vi "Main.vi"(8 "error in (no error)":errorcluster, 11 "StageSPIMBase in":refnum<class "StageSPIM.lvclass">) -> (0 "error out":errorcluster, 3 "component":refnum<class "StageSPIM.lvclass">)   [LabVIEW 2012, in "StageSPIM.lvclass"]
doc: "Main VI of the component."
uses:
  StageSPIM.lvclass
  <vilib>/Distrio/Murmex/Murmex/command_enum.ctl
  StageSPIM.lvclass/StageSPIM.ctl
  <vilib>/Distrio/Murmex/InitialiseMessage/InitialiseMessage.lvclass
  <vilib>/Distrio/Murmex/TerminateMessage/TerminateMessage.lvclass
  <vilib>/Distrio/Murmex/Murmex/update_cluster.ctl
  <vilib>/Distrio/Murmex/GenericMessage/GenericMessage.lvclass
  <vilib>/Distrio/Murmex/StopMessage/StopMessage.lvclass
  <vilib>/Distrio/Murmex/ConfigureMessage/ConfigureMessage.lvclass
  Global terminating.vi
  <vilib>/Distrio/Murmex/Murmex/Set configure at initialise.vi
  <vilib>/Distrio/Murmex/Murmex/Set log reference.vi
  <vilib>/Distrio/Murmex/Murmex/Set VI reference.vi
  <vilib>/Distrio/Murmex/Murmex/Get ID.vi
  <vilib>/Distrio/Murmex/Murmex/Set write log to disk.vi
  <vilib>/Distrio/Murmex/Murmex/Murmex.lvclass
  <vilib>/Distrio/Murmex/Message/Message.lvclass
panel:
  in  "Log position?":bool
  in  "button::stop":bool
  in  "button::configure":bool
  in  "button::quit":bool
  in  "Tab Control":enum32{"Main", "Debug"}(tab)
  in  "forwardFocus":bool
  in  "backFocus":bool
  in  "stepFocus":dbl[unit]
  out "currentFocus":dbl[unit]
  in  "speedFocus":dbl[unit]
  in  "targetFocus":dbl[unit]
  in  "forwardY":bool
  in  "backY":bool
  in  "stepY":dbl[unit]
  in  "forwardZ":bool
  in  "backZ":bool
  in  "stepZ":dbl[unit]
  in  "forwardX":bool
  in  "backX":bool
  in  "stepX":dbl[unit]
  in  "forwardA":bool
  in  "backA":bool
  in  "stepA":dbl[unit]
  out "currentA":dbl[unit]
  out "currentX":dbl[unit]
  out "currentY":dbl[unit]
  out "currentZ":dbl[unit]
  in  "speedZ":dbl[unit]
  in  "speedY":dbl[unit]
  in  "speedX":dbl[unit]
  in  "speedA":dbl[unit]
  in  "targetA":dbl[unit]
  in  "targetX":dbl[unit]
  in  "targetY":dbl[unit]
  in  "targetZ":dbl[unit]
  in  "button::send":bool
  out "log":string
  in  "command":T1
  in  "Generic command":string
  in  "ID":string="stage"
  out "terminate?":bool=TRUE
  # "Current\nposition"
  # "Target\nposition"
  # "Steps"
  # "Speed"
  # "A"
  # "X"
  # "Y"
  # "Z"
  # "Focus"
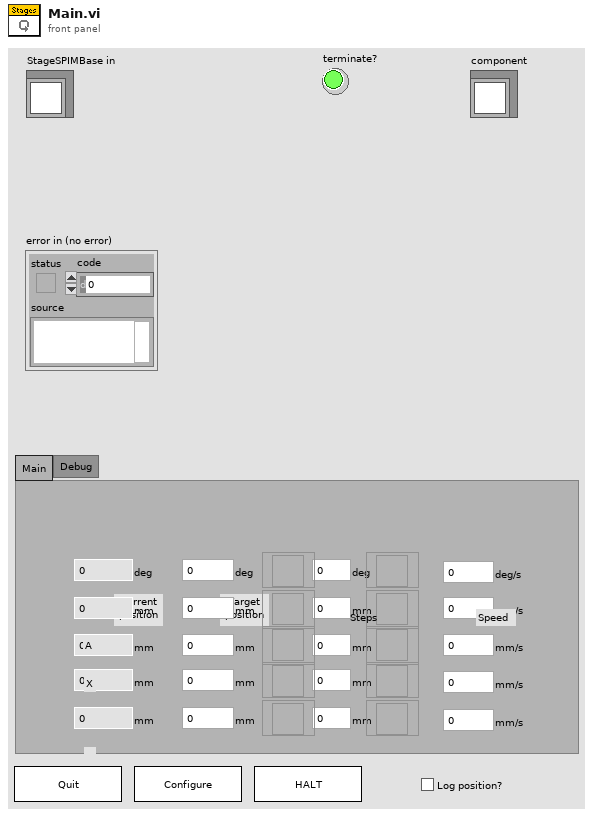
[diagram p1: front panel]
types:
  T1 = typedef "Murmex.lvlib/Murmex.lvclass/command_enum.ctl" = enum16{"null", "initialise", "reset", "terminate", "acknowledge", "update", "inspect", "inform", "proceed", "start", "stop", "fetch", "configure", "generic"}
  T2 = enum8{"Enabled", "Disabled", "Disabled and Grayed Out"}
  T3 = typedef "Murmex.lvlib/Murmex.lvclass/update_cluster.ctl" = cluster{"target ID":string, "key chains":string[], "values":variant[]}
  T4 = typedef "Murmex.lvlib/Murmex.lvclass/Event type enumerations.ctl" = enum16{"before", "after"}
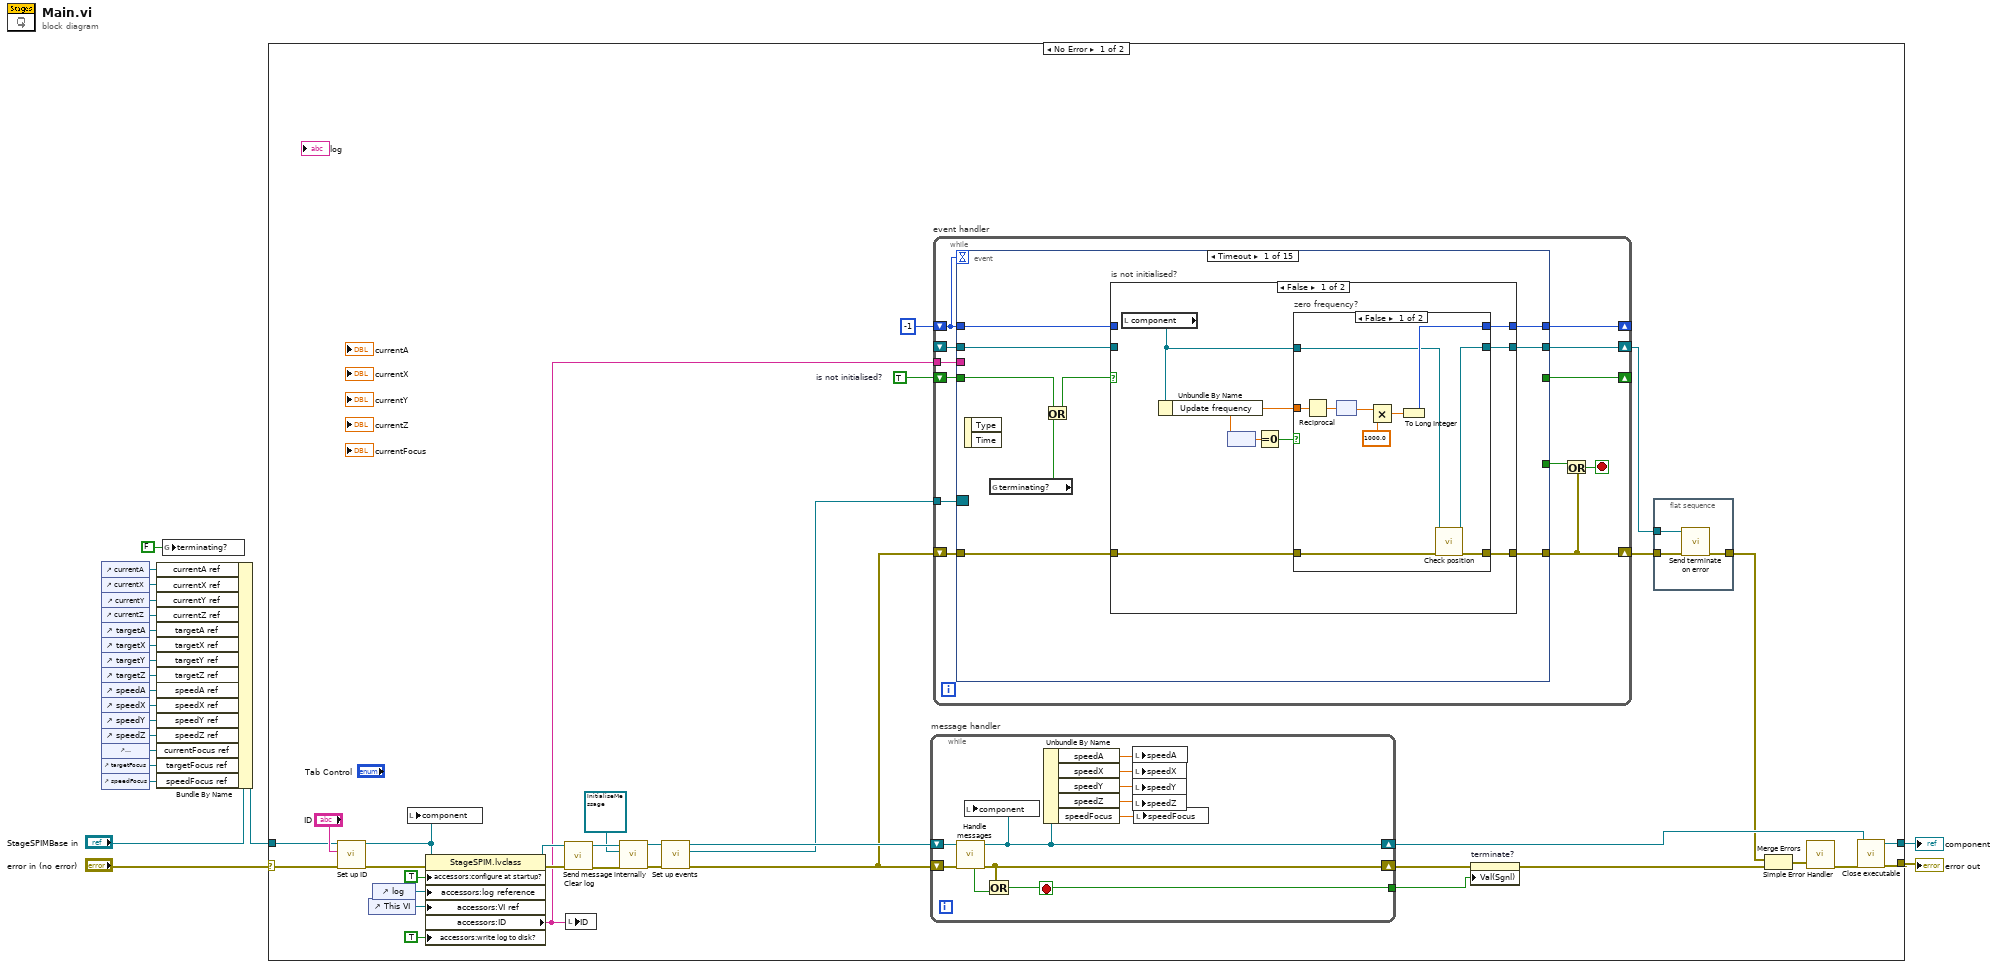
[diagram p0: block diagram]
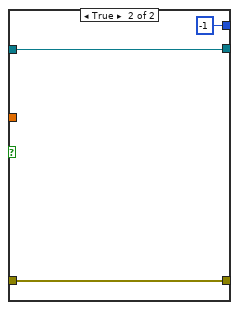
[diagram p2: hidden frame]
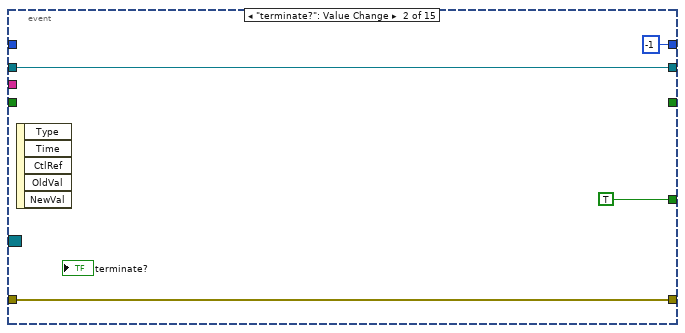
[diagram p4: hidden frame]
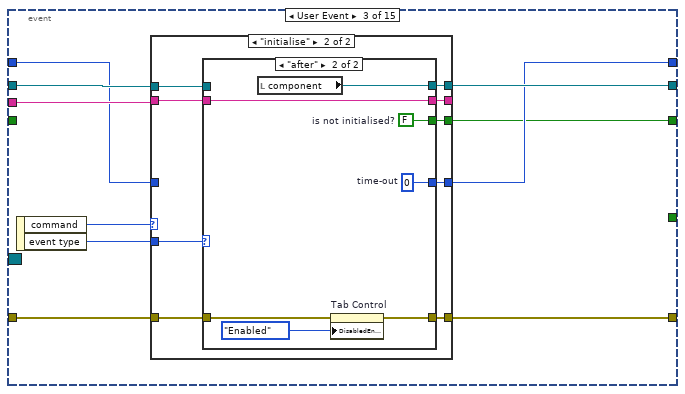
[diagram p5: hidden frame]
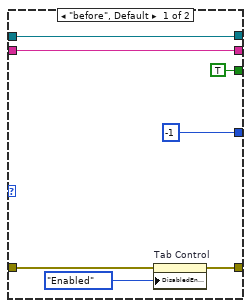
[diagram p7: hidden frame]
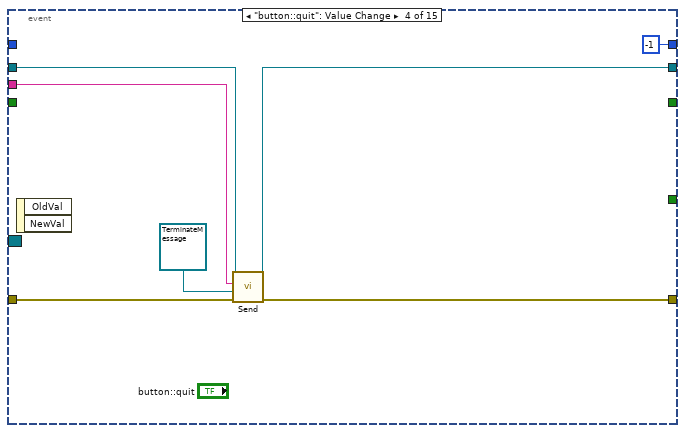
[diagram p8: hidden frame]
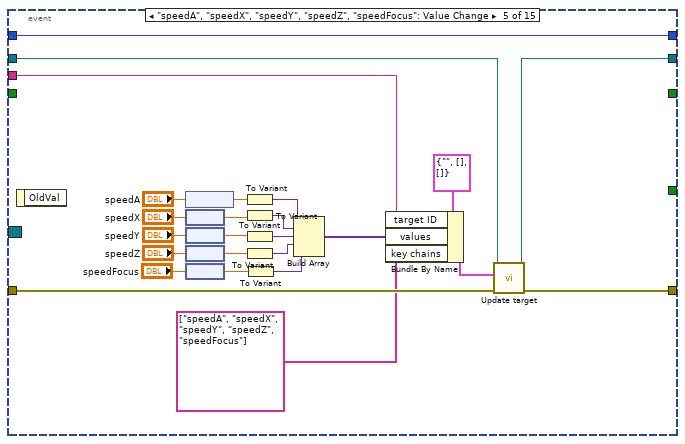
[diagram p9: hidden frame]
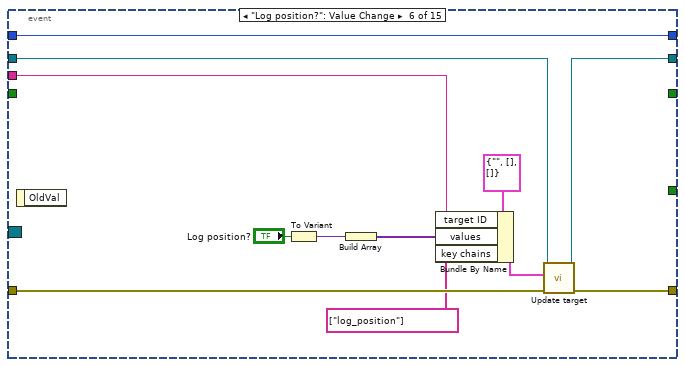
[diagram p10: hidden frame]
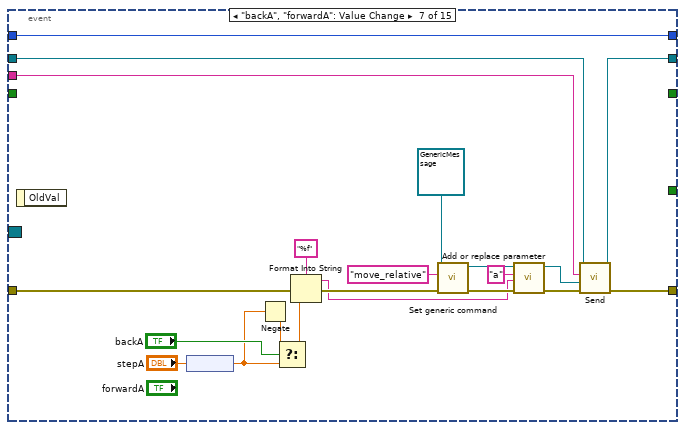
[diagram p11: hidden frame]
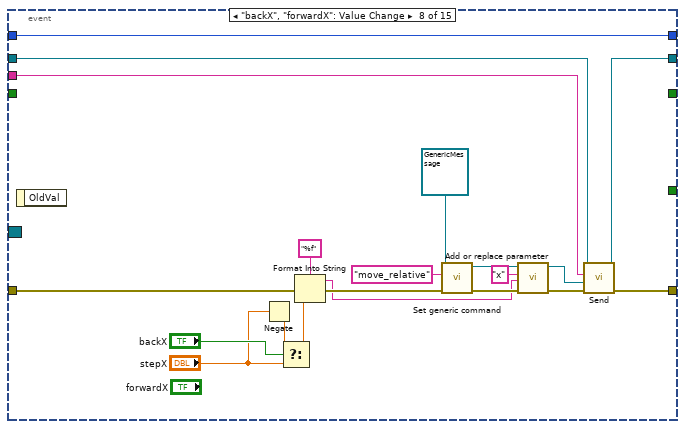
[diagram p12: hidden frame]
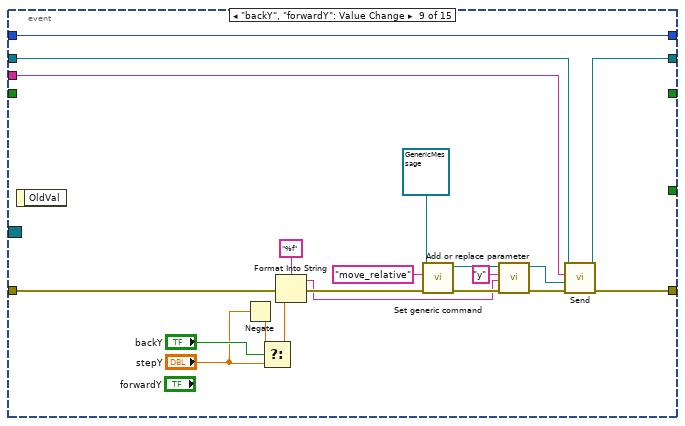
[diagram p13: hidden frame]
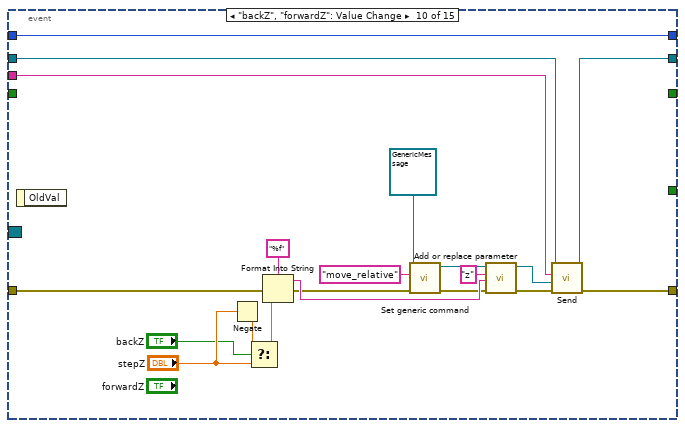
[diagram p14: hidden frame]
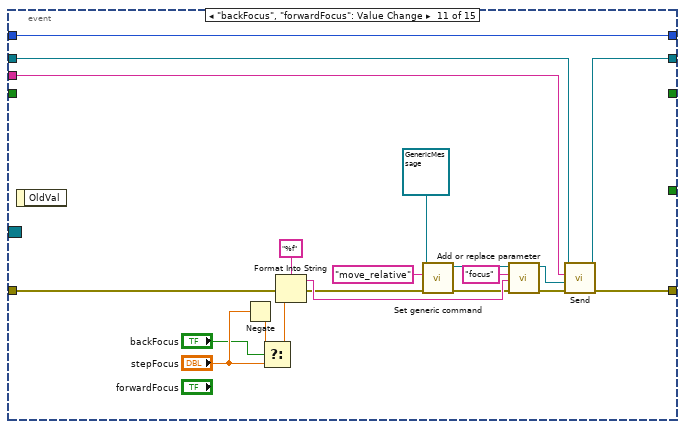
[diagram p15: hidden frame]
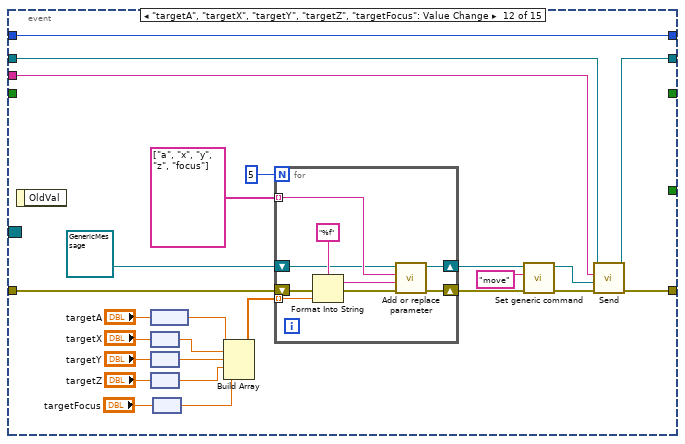
[diagram p16: hidden frame]
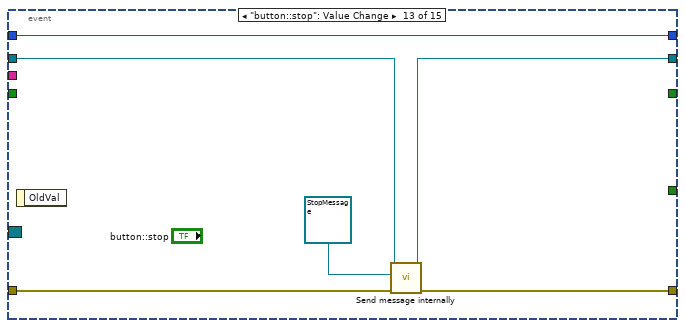
[diagram p17: hidden frame]
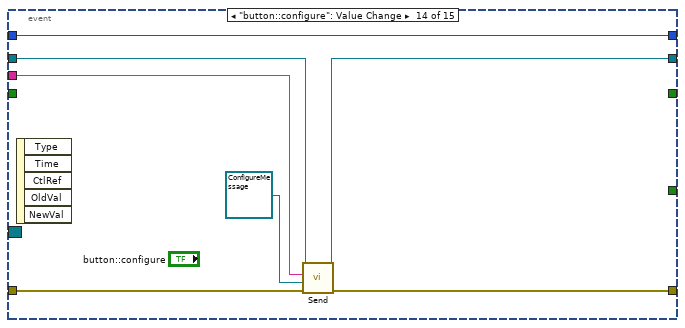
[diagram p18: hidden frame]
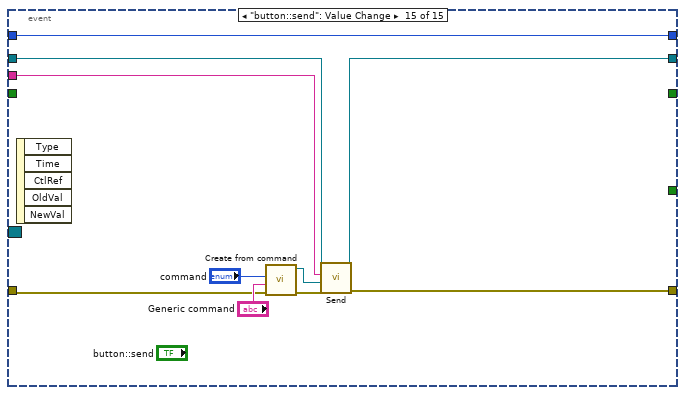
[diagram p19: hidden frame]
diagram:
  n1 = control-ref of="currentA"() -> (w16:refnum<vi>)
  n2 = control-ref of="currentX"() -> (w15:refnum<vi>)
  n3 = control-ref of="currentY"() -> (w14:refnum<vi>)
  n4 = control-ref of="currentZ"() -> (w13:refnum<vi>)
  n5 = control-ref of="targetA"() -> (w12:refnum<vi>)
  n6 = control-ref of="targetX"() -> (w11:refnum<vi>)
  n7 = control-ref of="targetY"() -> (w10:refnum<vi>)
  n8 = control-ref of="targetZ"() -> (w9:refnum<vi>)
  n9 = control-ref of="speedA"() -> (w8:refnum<vi>)
  n10 = control-ref of="speedX"() -> (w7:refnum<vi>)
  n11 = control-ref of="speedY"() -> (w6:refnum<vi>)
  n12 = control-ref of="speedZ"() -> (w5:refnum<vi>)
  n13 = control-ref of="currentFocus"() -> (w4:refnum<vi>)
  n14 = control-ref of="targetFocus"() -> (w3:refnum<vi>)
  n15 = control-ref of="speedFocus"() -> (w2:refnum<vi>)
  n16 = Bundle By Name(cluster="StageSPIMBase in", "currentA ref"=w16, "currentX ref"=w15, "currentY ref"=w14, "currentZ ref"=w13, "targetA ref"=w12, "targetX ref"=w11, "targetY ref"=w10, "targetZ ref"=w9, "speedA ref"=w8, "speedX ref"=w7, "speedY ref"=w6, "speedZ ref"=w5, "currentFocus ref"=w4, "targetFocus ref"=w3, "speedFocus ref"=w2) -> (w19:refnum<class "StageSPIM.lvclass">)
  n17 = global write "Global terminating.vi" "terminating?"(FALSE ("terminating?")) -> ()
  n18 = case shown="No Error" "error in (no error)" {
    selector: "error in (no error)" -> [w53 w357]
    tunnel: w19 -> [w52 w358]
    tunnel: [w37 w357] -> w18
    tunnel: [w35 w358] -> w17
    frame No Error {
      w27 = TRUE  # is not initialised?
      n19 = call <vilib>:"Set up ID.vi"("error in (no error)"=w53, "component ID"="ID", "MurmexBase in"=w52) -> ("error out"=w51:errorcluster, "MurmexBase out"=w28:refnum<class "StageSPIM.lvclass">)  [unwired: 6 in, 1 out]
      n20 = control-ref of="This VI"() -> (w48:refnum<vi>)
      n21 = control-ref of="log"() -> (w49:refnum<vi>)
      n22 = local write "component"(w28) -> ()
      n23 = property class="StageSPIM.lvclass"(reference=w28, error in=w51, "accessors:configure at startup?"=TRUE ("configure at startup?"), "accessors:log reference"=w49, "accessors:VI ref"=w48, "accessors:write log to disk?"=TRUE ("write log to disk?")) -> (reference out=w46:refnum<class "StageSPIM.lvclass">, error out=w47:errorcluster, "accessors:ID"=w29:string)
      n24 = call <vilib>:"Clear log.vi"("error in (no error)"=w47, "MurmexBase in"=w46) -> ("error out"=w45:errorcluster, "MurmexBase out"=w44:refnum<class "StageSPIM.lvclass">)  [unwired: 8 in]
      n25 = local write "ID"(w29) -> ()
      n26 = call <vilib>:"Send message internally.vi"("error in (no error)"=w45, "Message"=refnum<class "InitialiseMessage.lvclass"> refnum ("Distrio Murmex 1.1:InitialiseMessage"), "Murmex in"=w44) -> ("error out"=w42:errorcluster, "Murmex out"=w41:refnum<class "StageSPIM.lvclass">)  [unwired: 7 in]
      n27 = call <vilib>:"Set up events.vi"("error in (no error)"=w42, "MurmexBase in"=w41) -> ("error out"=w34:errorcluster, "Event Registration Refnum"=w33:refnum<event-registration>, "MurmexBase out"=w40:refnum<class "StageSPIM.lvclass">)  [unwired: 7 in]
      n28 = while "message handler" {
        shift-right: [w354] -> w26
        shift-left: w34 -> [w356]
        shift-right: [w351] -> w36
        shift-left: w40 -> [w355]
        tunnel: [w352] -> w22
        stop <- w352 stop-if-true
        n29 = call <vilib>:"Handle messages.vi"("error in (no error)"=w356, "Murmex in"=w355) -> ("error out"=w354:errorcluster, "Murmex out"=w351:refnum<class "StageSPIM.lvclass">, "terminated?"=w353:bool)  [unwired: 7 in]
        n30 = local write "component"(w351) -> ()
        n31 = Or(x=w354, y=w353) -> (x .or. y?=w352:bool)
        n32 = Unbundle By Name(w351) -> ("speedA"=w350:dbl[unit], "speedX"=w349:dbl[unit], "speedY"=w348:dbl[unit], "speedZ"=w347:dbl[unit], "speedFocus"=w346:dbl[unit])
        n33 = local write "speedA"(w350) -> ()
        n34 = local write "speedX"(w349) -> ()
        n35 = local write "speedY"(w348) -> ()
        n36 = local write "speedZ"(w347) -> ()
        n37 = local write "speedFocus"(w346) -> ()
      }
      n38 = while "event handler" {
        shift-right: [w60] -> w31
        shift-left: w34 -> [w69]
        tunnel: w33 -> [w68]
        shift-right: [w66] -> _
        shift-left: -1 -> [w67]
        shift-right: [w63] -> w24
        shift-left: _ -> [w62]
        shift-right: [w58] -> _
        shift-left: w27 -> [w59]
        tunnel: w29 -> [w64]
        stop <- w65 stop-if-true
        n39 = event shown="[0] Timeout" {
          selector: w68 -> [_ _ _ _ _ _ _ _ _ _ _ _ _ _ _]
          dyn-events: _ -> [_ _ _ _ _ _ _ _ _ _ _ _ _ _ _]
          timeout: w67 -> [_ _ _ _ _ _ _ _ _ _ _ _ _ _ _]
          tunnel: w69 -> [w77 w106 w116 w149 w174 w184 w207 w210 w232 w252 w273 w292 w328 w335 w341]
          tunnel: w67 -> [w73 _ w108 _ w159 w181 w208 w209 w231 w253 w269 w308 w326 w329 w337]
          tunnel: [w78 -1 ("time-out") w109 -1 ("time-out") w159 w181 w208 w209 w231 w253 w269 w308 w326 w329 w337] -> w66
          tunnel: [w76 w106 w110 w148 w173 w185 w197 w216 w236 w255 w276 w312 w324 w334 w340] -> w60
          tunnel: w64 -> [_ _ w113 w145 w172 w180 w194 w213 w233 w254 w270 w309 _ w332 w336]
          tunnel: w62 -> [w74 w104 w112 w147 w171 w183 w196 w214 w234 w249 w272 w310 w327 w331 w339]
          tunnel: [w75 w104 w111 w146 w170 w182 w195 w215 w235 w256 w271 w311 w325 w330 w338] -> w63
          tunnel: [_ TRUE _ _ _ _ _ _ _ _ _ _ _ _ _] -> w61
          tunnel: w59 -> [w72 _ _ _ _ _ _ _ _ _ _ _ _ _ _]
          tunnel: [_ _ w107 _ _ _ _ _ _ _ _ _ _ _ _] -> w58
          event Timeout {
            n40 = event-data() -> ()  [unwired: 1 in, 2 out]
            n41 = global read "Global terminating.vi" "terminating?"() -> (w70:bool)
            n42 = Or(x=w72, y=w70) -> (x .or. y?=w71:bool)
            n43 = case "is not initialised?" shown="False" w71 {
              tunnel: [w86 w100] -> w78
              tunnel: w77 -> [w85 w102]
              tunnel: [w84 w102] -> w76
              tunnel: [w83 w101] -> w75
              tunnel: w74 -> [_ w101]
              tunnel: w73 -> [_ w100]
              frame False {
                n44 = local read "component"() -> (w79:refnum<class "StageSPIM.lvclass">)
                n45 = Unbundle By Name(w79) -> ("Update frequency"=w82:dbl[unit])
                n46 = node(w82) -> (w81:dbl)
                n47 = Equal To 0?(x=w81) -> (x = 0?=w80:bool)
                n48 = case "zero frequency?" shown="False" w80 {
                  tunnel: [w92 -1] -> w86
                  tunnel: w85 -> [w90 w98]
                  tunnel: [w89 w98] -> w84
                  tunnel: w79 -> [w88 w99]
                  tunnel: [w87 w99] -> w83
                  tunnel: w82 -> [w91 _]
                  frame False {
                    n49 = Reciprocal(x=w91) -> (1/x=w96:dbl[unit])
                    n50 = node(w96) -> (w94:dbl)
                    n51 = Multiply(x=w94, y=1000.0) -> (x*y=w93:dbl)
                    n52 = To Long Integer(number=w93) -> (32bit integer=w92:i32)
                    n53 = call-dynamic "Check position.vi"("error in (no error)"=w90, "StageSPIM in"=w88) -> ("error out"=w89:errorcluster, "StageSPIM out"=w87:refnum<class "StageSPIM.lvclass">)  [unwired: 8 in]
                  }
                  frame True {
                  }
                }
              }
              frame True {
              }
            }
          }
          event "terminate?": Value Change {
            n54 = event-data() -> ()  [unwired: 1 in, 5 out]
          }
          event User Event {
            n55 = event-data() -> ("command"=w115:T1, "event type"=w114:T4)  [unwired: 1 in]
            n56 = case shown="\"initialise\"" w115 {
              tunnel: w116 -> [w118 w129]
              tunnel: [w118 w128] -> w110
              tunnel: w113 -> [w120 w127]
              tunnel: [w119 w126] -> w111
              tunnel: w112 -> [w119 w125]
              tunnel: [w120 w124] -> _
              tunnel: w114 -> [_ w123]
              tunnel: [w117 w122] -> w109
              tunnel: w108 -> [w117 _]
              tunnel: [_ w121] -> w107
              frame "null", Default {
              }
              frame "initialise" {
                n57 = case shown="\"after\"" w123 {
                  tunnel: [w135 w142] -> w128
                  tunnel: w129 -> [w136 w143]
                  tunnel: w127 -> [w133 w139]
                  tunnel: [w132 w141] -> w126
                  tunnel: w125 -> [w132 _]
                  tunnel: [w133 w139] -> w124
                  tunnel: [-1 w138] -> w122
                  tunnel: [TRUE ("is not initialised?") w137] -> w121
                  frame "before", Default {
                    n58 = property on="Tab Control" class="TabCtl (strict)"(error in=w136, "DisabledEnum"=T2."Enabled" ("Disabled")) -> (error out=w135:errorcluster)  [unwired: 1 in, 1 out]
                  }
                  frame "after" {
                    w137 = FALSE  # is not initialised?
                    w138 = 0  # time-out
                    n59 = local read "component"() -> (w141:refnum<class "StageSPIM.lvclass">)
                    n60 = property on="Tab Control" class="TabCtl (strict)"(error in=w143, "DisabledEnum"=T2."Enabled" ("Disabled")) -> (error out=w142:errorcluster)  [unwired: 1 in, 1 out]
                  }
                }
              }
            }
          }
          event "button::quit": Value Change {
            n61 = event-data() -> ()  [unwired: 1 in, 2 out]
            n62 = call <vilib>:"Send.vi"("error in (no error)"=w149, "Message"=refnum<class "TerminateMessage.lvclass"> refnum ("Murmex.lvlib:TerminateMessage"), "recipient"=w145, "Murmex in"=w147) -> ("error out"=w148:errorcluster, "Murmex out"=w146:refnum<class "StageSPIM.lvclass">)  [unwired: 6 in]
          }
          event "speedA", "speedX", "speedY", "speedZ", "speedFocus": Value Change {
            n63 = event-data() -> ()  [unwired: 1 in, 1 out]
            n64 = node("speedA") -> (w158:dbl)
            n65 = node("speedX") -> (w155:dbl)
            n66 = node("speedY") -> (w156:dbl)
            n67 = node("speedZ") -> (w157:dbl)
            n68 = node("speedFocus") -> (w153:dbl)
            n69 = To Variant(anything=w158) -> (Variant=w165:variant)
            n70 = To Variant(anything=w155) -> (Variant=w164:variant)
            n71 = To Variant(anything=w156) -> (Variant=w163:variant)
            n72 = To Variant(anything=w157) -> (Variant=w162:variant)
            n73 = To Variant(anything=w153) -> (Variant=w152:variant)
            n74 = Build Array(w165, w164, w163, w162, w152) -> (w161:variant[])
            n75 = Bundle By Name(cluster=T3 {"target ID"="", "key chains"=[], "values"=[]} ("update cluster"), "target ID"=w172, "values"=w161, "key chains"=string[] ["speedA", "speedX", "speedY", "speedZ", "speedFocus"]) -> (w151:T3)
            n76 = call <vilib>:"Update target.vi"("error in (no error)"=w174, "update cluster"=w151, "MurmexBase in"=w171) -> ("error out"=w173:errorcluster, "MurmexBase out"=w170:refnum<class "StageSPIM.lvclass">)  [unwired: 7 in]
          }
          event "Log position?": Value Change {
            n77 = event-data() -> ()  [unwired: 1 in, 1 out]
            n78 = To Variant(anything="Log position?") -> (Variant=w178:variant)
            n79 = Build Array(w178) -> (w177:variant[])
            n80 = Bundle By Name(cluster=T3 {"target ID"="", "key chains"=[], "values"=[]} ("update cluster"), "target ID"=w180, "values"=w177, "key chains"=string[] ["log_position"]) -> (w186:T3)
            n81 = call <vilib>:"Update target.vi"("error in (no error)"=w184, "update cluster"=w186, "MurmexBase in"=w183) -> ("error out"=w185:errorcluster, "MurmexBase out"=w182:refnum<class "StageSPIM.lvclass">)  [unwired: 7 in]
          }
          event "backA", "forwardA": Value Change {
            n82 = event-data() -> ()  [unwired: 1 in, 1 out]
            n83 = node("stepA") -> (w188:dbl)
            n84 = Negate(x=w188) -> (-x=w201:dbl)
            n85 = Select(t=w201, s="backA", f=w188) -> (s? t:f=w190:dbl)
            n86 = Format Into String(format string="%f", error in=w207, w190) -> (resulting string=w191:string, error out=w198:errorcluster)  [unwired: 1 in]
            n87 = call <vilib>:"Set generic command.vi"("error in (no error)"=w198, "generic command"="move_relative", "GenericMessage in"=refnum<class "GenericMessage.lvclass"> refnum ("Distrio Murmex 1.1:GenericMessage")) -> ("error out"=w205:errorcluster, "GenericMessage out"=w203:refnum<class "GenericMessage.lvclass">)  [unwired: 7 in]
            n88 = call <vilib>:"Add or replace parameter.vi"("error in (no error)"=w205, "value"=w191, "name"="a", "Message in"=w203) -> ("error out"=w204:errorcluster, "Message out"=w192:refnum<class "GenericMessage.lvclass">)  [unwired: 6 in]
            n89 = call <vilib>:"Send.vi"("error in (no error)"=w204, "Message"=w192, "recipient"=w194, "Murmex in"=w196) -> ("error out"=w197:errorcluster, "Murmex out"=w195:refnum<class "StageSPIM.lvclass">)  [unwired: 6 in]
          }
          event "backX", "forwardX": Value Change {
            n90 = event-data() -> ()  [unwired: 1 in, 1 out]
            n91 = Negate(x="stepX") -> (-x=w223:dbl[unit])
            n92 = Select(t=w223, s="backX", f="stepX") -> (s? t:f=w218:dbl[unit])
            n93 = Format Into String(format string="%f", error in=w210, w218) -> (resulting string=w219:string, error out=w222:errorcluster)  [unwired: 1 in]
            n94 = call <vilib>:"Set generic command.vi"("error in (no error)"=w222, "generic command"="move_relative", "GenericMessage in"=refnum<class "GenericMessage.lvclass"> refnum ("Distrio Murmex 1.1:GenericMessage")) -> ("error out"=w227:errorcluster, "GenericMessage out"=w225:refnum<class "GenericMessage.lvclass">)  [unwired: 7 in]
            n95 = call <vilib>:"Add or replace parameter.vi"("error in (no error)"=w227, "value"=w219, "name"="x", "Message in"=w225) -> ("error out"=w226:errorcluster, "Message out"=w220:refnum<class "GenericMessage.lvclass">)  [unwired: 6 in]
            n96 = call <vilib>:"Send.vi"("error in (no error)"=w226, "Message"=w220, "recipient"=w213, "Murmex in"=w214) -> ("error out"=w216:errorcluster, "Murmex out"=w215:refnum<class "StageSPIM.lvclass">)  [unwired: 6 in]
          }
          event "backY", "forwardY": Value Change {
            n97 = event-data() -> ()  [unwired: 1 in, 1 out]
            n98 = Negate(x="stepY") -> (-x=w243:dbl[unit])
            n99 = Select(t=w243, s="backY", f="stepY") -> (s? t:f=w238:dbl[unit])
            n100 = Format Into String(format string="%f", error in=w232, w238) -> (resulting string=w239:string, error out=w242:errorcluster)  [unwired: 1 in]
            n101 = call <vilib>:"Set generic command.vi"("error in (no error)"=w242, "generic command"="move_relative", "GenericMessage in"=refnum<class "GenericMessage.lvclass"> refnum ("Distrio Murmex 1.1:GenericMessage")) -> ("error out"=w247:errorcluster, "GenericMessage out"=w245:refnum<class "GenericMessage.lvclass">)  [unwired: 7 in]
            n102 = call <vilib>:"Add or replace parameter.vi"("error in (no error)"=w247, "value"=w239, "name"="y", "Message in"=w245) -> ("error out"=w246:errorcluster, "Message out"=w240:refnum<class "GenericMessage.lvclass">)  [unwired: 6 in]
            n103 = call <vilib>:"Send.vi"("error in (no error)"=w246, "Message"=w240, "recipient"=w233, "Murmex in"=w234) -> ("error out"=w236:errorcluster, "Murmex out"=w235:refnum<class "StageSPIM.lvclass">)  [unwired: 6 in]
          }
          event "backZ", "forwardZ": Value Change {
            n104 = event-data() -> ()  [unwired: 1 in, 1 out]
            n105 = Negate(x="stepZ") -> (-x=w262:dbl[unit])
            n106 = Select(t=w262, s="backZ", f="stepZ") -> (s? t:f=w267:dbl[unit])
            n107 = Format Into String(format string="%f", error in=w252, w267) -> (resulting string=w266:string, error out=w263:errorcluster)  [unwired: 1 in]
            n108 = call <vilib>:"Set generic command.vi"("error in (no error)"=w263, "generic command"="move_relative", "GenericMessage in"=refnum<class "GenericMessage.lvclass"> refnum ("Distrio Murmex 1.1:GenericMessage")) -> ("error out"=w258:errorcluster, "GenericMessage out"=w260:refnum<class "GenericMessage.lvclass">)  [unwired: 7 in]
            n109 = call <vilib>:"Add or replace parameter.vi"("error in (no error)"=w258, "value"=w266, "name"="z", "Message in"=w260) -> ("error out"=w259:errorcluster, "Message out"=w265:refnum<class "GenericMessage.lvclass">)  [unwired: 6 in]
            n110 = call <vilib>:"Send.vi"("error in (no error)"=w259, "Message"=w265, "recipient"=w254, "Murmex in"=w249) -> ("error out"=w255:errorcluster, "Murmex out"=w256:refnum<class "StageSPIM.lvclass">)  [unwired: 6 in]
          }
          event "backFocus", "forwardFocus": Value Change {
            n111 = event-data() -> ()  [unwired: 1 in, 1 out]
            n112 = Negate(x="stepFocus") -> (-x=w282:dbl[unit])
            n113 = Select(t=w282, s="backFocus", f="stepFocus") -> (s? t:f=w287:dbl[unit])
            n114 = Format Into String(format string="%f", error in=w273, w287) -> (resulting string=w286:string, error out=w283:errorcluster)  [unwired: 1 in]
            n115 = call <vilib>:"Set generic command.vi"("error in (no error)"=w283, "generic command"="move_relative", "GenericMessage in"=refnum<class "GenericMessage.lvclass"> refnum ("Distrio Murmex 1.1:GenericMessage")) -> ("error out"=w278:errorcluster, "GenericMessage out"=w280:refnum<class "GenericMessage.lvclass">)  [unwired: 7 in]
            n116 = call <vilib>:"Add or replace parameter.vi"("error in (no error)"=w278, "value"=w286, "name"="focus", "Message in"=w280) -> ("error out"=w279:errorcluster, "Message out"=w285:refnum<class "GenericMessage.lvclass">)  [unwired: 6 in]
            n117 = call <vilib>:"Send.vi"("error in (no error)"=w279, "Message"=w285, "recipient"=w270, "Murmex in"=w272) -> ("error out"=w276:errorcluster, "Murmex out"=w271:refnum<class "StageSPIM.lvclass">)  [unwired: 6 in]
          }
          event "targetA", "targetX", "targetY", "targetZ", "targetFocus": Value Change {
            n118 = event-data() -> ()  [unwired: 1 in, 1 out]
            n119 = node("targetA") -> (w295:dbl)
            n120 = node("targetX") -> (w299:dbl)
            n121 = node("targetY") -> (w296:dbl)
            n122 = node("targetZ") -> (w291:dbl)
            n123 = node("targetFocus") -> (w289:dbl)
            n124 = Build Array(w295, w299, w296, w291, w289) -> (w293:dbl[])
            n125 = for {
              N: 5 -> [_]
              shift-right: [w320] -> w305
              shift-left: w292 -> [w319]
              tunnel: string[] ["a", "x", "y", "z", "focus"] -> [w318] mode=indexing
              shift-right: [w316] -> w301
              shift-left: refnum<class "GenericMessage.lvclass"> refnum ("Distrio Murmex 1.1:GenericMessage") -> [w317]
              tunnel: w293 -> [w315] mode=indexing
              n126 = Format Into String(format string="%f", error in=w319, w315) -> (resulting string=w314:string, error out=w321:errorcluster)  [unwired: 1 in]
              n127 = call <vilib>:"Add or replace parameter.vi"("error in (no error)"=w321, "value"=w314, "name"=w318, "Message in"=w317) -> ("error out"=w320:errorcluster, "Message out"=w316:refnum<class "GenericMessage.lvclass">)  [unwired: 6 in]
            }
            n128 = call <vilib>:"Set generic command.vi"("error in (no error)"=w305, "generic command"="move", "GenericMessage in"=w301) -> ("error out"=w307:errorcluster, "GenericMessage out"=w306:refnum<class "GenericMessage.lvclass">)  [unwired: 7 in]
            n129 = call <vilib>:"Send.vi"("error in (no error)"=w307, "Message"=w306, "recipient"=w309, "Murmex in"=w310) -> ("error out"=w312:errorcluster, "Murmex out"=w311:refnum<class "StageSPIM.lvclass">)  [unwired: 6 in]
          }
          event "button::stop": Value Change {
            n130 = event-data() -> ()  [unwired: 1 in, 1 out]
            n131 = call <vilib>:"Send message internally.vi"("error in (no error)"=w328, "Message"=refnum<class "StopMessage.lvclass"> refnum ("Distrio Murmex 1.5:StopMessage"), "Murmex in"=w327) -> ("error out"=w324:errorcluster, "Murmex out"=w325:refnum<class "StageSPIM.lvclass">)  [unwired: 7 in]
          }
          event "button::configure": Value Change {
            n132 = event-data() -> ()  [unwired: 1 in, 5 out]
            n133 = call <vilib>:"Send.vi"("error in (no error)"=w335, "Message"=refnum<class "ConfigureMessage.lvclass"> refnum ("Distrio Murmex 1.1:ConfigureMessage"), "recipient"=w332, "Murmex in"=w331) -> ("error out"=w334:errorcluster, "Murmex out"=w330:refnum<class "StageSPIM.lvclass">)  [unwired: 6 in]
          }
          event "button::send": Value Change {
            n134 = event-data() -> ()  [unwired: 1 in, 5 out]
            n135 = call <vilib>:"Create from command.vi"("error in (no error)"=w341, "generic command"="Generic command", "command"="command") -> ("error out"=w343:errorcluster, "Message out"=w344:refnum<class "Message.lvclass">)  [unwired: 7 in]
            n136 = call <vilib>:"Send.vi"("error in (no error)"=w343, "Message"=w344, "recipient"=w336, "Murmex in"=w339) -> ("error out"=w340:errorcluster, "Murmex out"=w338:refnum<class "StageSPIM.lvclass">)  [unwired: 6 in]
          }
        }
        n137 = Or(x=w61, y=w60) -> (x .or. y?=w65:bool)
      }
      n138 = property on="terminate?" class="Bool (strict)"(error in=w26, "Val(Sgnl)"=w22) -> (error out=w25:errorcluster)  [unwired: 1 in, 1 out]
      n139 = flat-sequence {
        tunnel: w31 -> [w57]
        tunnel: [w56] -> w30
        tunnel: w24 -> [w55]
        frame #0 {
          n140 = call <vilib>:"Send terminate on error.vi"("error in (no error)"=w57, "Murmex in"=w55) -> ("error out"=w56:errorcluster)  [unwired: 8 in, 1 out]
        }
      }
      n141 = Merge Errors(w30, w25) -> (w39:errorcluster)
      n142 = call <vilib>:"Simple Error Handler.vi"("error in (no error)"=w39) -> ("error out"=w38:errorcluster)  [unwired: 4 in, 4 out]
      n143 = call <vilib>:"Close executable.vi"("error in (no error)"=w38, "MurmexBase in"=w36) -> ("error out"=w37:errorcluster, "MurmexBase out"=w35:refnum<class "StageSPIM.lvclass">)  [unwired: 8 in]
    }
    frame Error {
    }
  }
  "error out" <- w18
  "component" <- w17
